vi "Initialize Title Bar.vi"(7 "QRD":T1, 8 "error in":errorcluster) -> (0 "error out":errorcluster, 5 "QRD Out":T1)   [LabVIEW 2025]
uses:
  Builds/Queue Wrappers.lvlibp/Q Packet.ctl
  Builds/Queue Wrappers.lvlibp
  Controls/Queues-Refs-Data.ctl
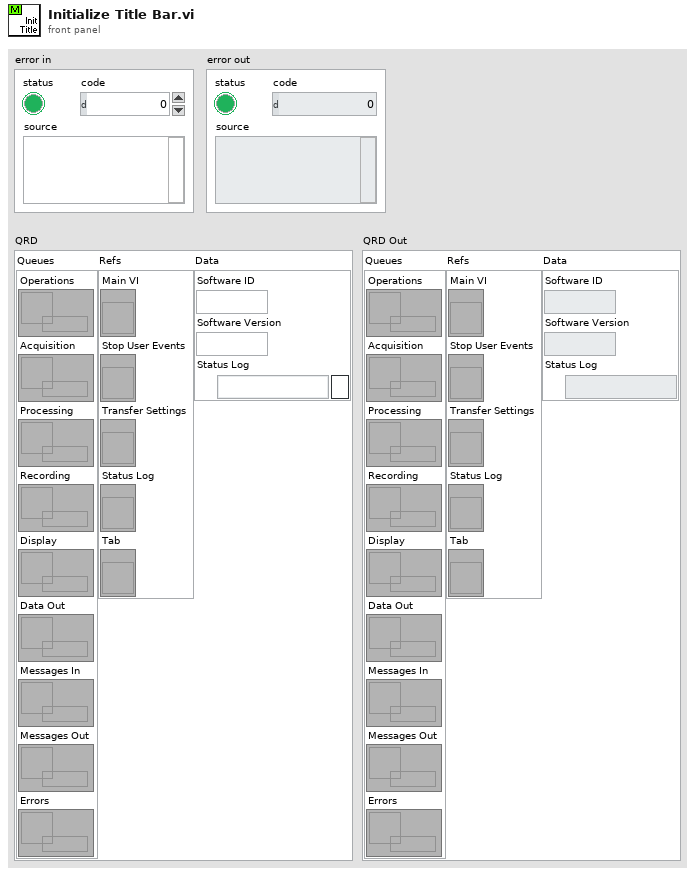
[diagram p1: front panel]
types:
  T1 = typedef "Queues-Refs-Data.ctl" = cluster{"Queues":cluster{"Operations":refnum<queue>, "Acquisition":refnum<queue>, "Processing":refnum<queue>, "Recording":refnum<queue>, "Display":refnum<queue>, "Data Out":refnum<queue>, "Messages In":refnum<queue>, "Messages Out":refnum<queue>, "Errors":refnum<queue>}, "Refs":cluster{"Main VI":refnum<vi>, "Stop User Events":refnum<vi>, "Transfer Settings":refnum<vi>, "Status Log":refnum<vi>, "Tab":refnum<vi>}, "Data":cluster{"Software ID":string, "Software Version":string, "Status Log":path}}
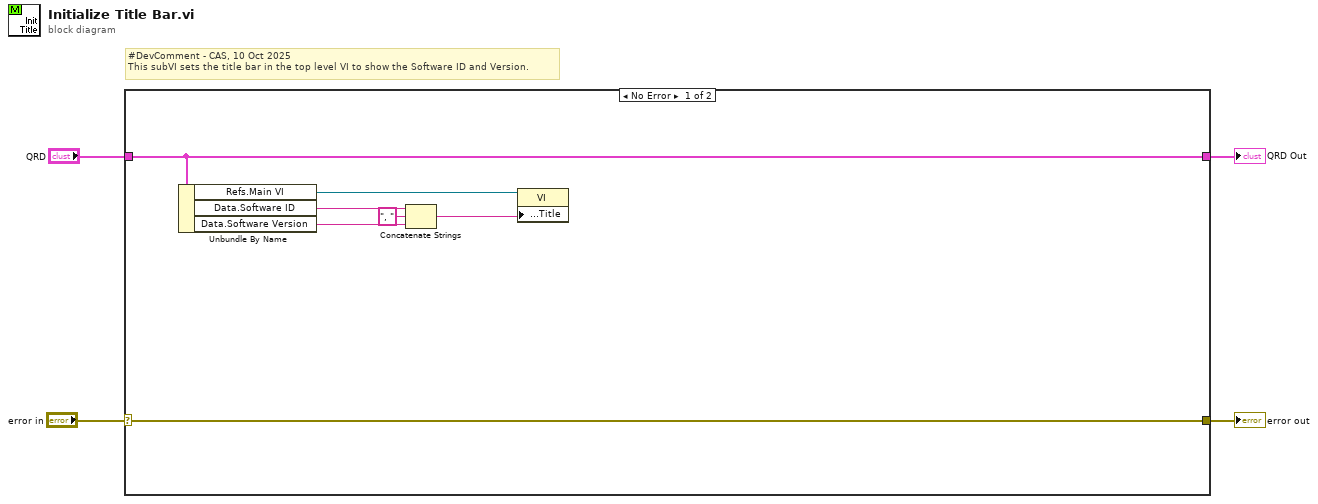
[diagram p0: block diagram]
diagram:
  # "#DevComment - CAS, 10 Oct 2025\nThis subVI sets the title bar in the top level VI to show the Software ID and Version."
  n1 = case shown="No Error" "error in" {
    selector: "error in" -> [w5 w13]
    tunnel: "QRD" -> [w6 w12]
    tunnel: [w6 w12] -> w3
    tunnel: [w5 w13] -> w1
    frame No Error {
      n2 = Unbundle By Name(w6) -> ("Refs.Main VI"=w11:refnum<vi>, "Data.Software ID"=w10:string, "Data.Software Version"=w9:string)
      n3 = Concatenate Strings(w10, ", " ("string"), w9) -> (w7:string)
      n4 = property class="VI"(reference=w11, "Front Panel.Title"=w7) -> ()  [unwired: 1 in, 2 out]
    }
    frame Error {
    }
  }
  "error out" <- w1
  "QRD Out" <- w3
